vi "Stop.vi"(8 "error in (no error)":errorcluster, 11 "XNET Base CFG in":refnum<class "XNET Base CFG.lvclass">) -> (0 "error out":errorcluster, 3 "XNET Base CFG out":refnum<class "XNET Base CFG.lvclass">)   [LabVIEW 2023, in "XNET Base CFG.lvclass"]
uses:
  XNET Base CFG.lvclass
  XNET Base CFG.lvclass/XNET Base CFG.ctl
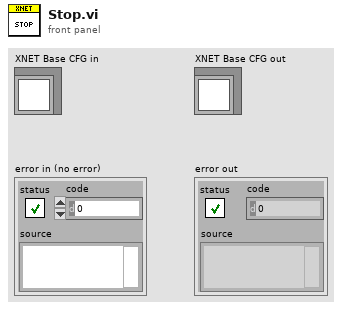
[diagram p1: front panel]
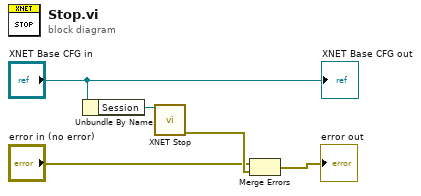
[diagram p0: block diagram]
diagram:
  n1 = Unbundle By Name("XNET Base CFG in") -> ("Session"=w5:refnum<k21>)
  n2 = call <vilib>:"XNET Stop.vi"("session in"=w5) -> ("error out"=w2:errorcluster)  [unwired: 13 in, 1 out]
  n3 = Merge Errors("error in (no error)", w2) -> (→"error out":errorcluster)
  "XNET Base CFG out" <- "XNET Base CFG in"
